vi "Write Data to HW.vi"(11 "CD in":refnum<class "Template.lvclass">) -> (0 "error out":errorcluster, 3 "CD out":refnum<class "Template.lvclass">)   [LabVIEW 2026, in "Template Plugin.lvlib" / "Template.lvclass"]
uses:
  Template.lvclass
  Template.lvclass/Template.ctl
  <userlib>/CustomDeviceInterfaces_v1.lvlibp/custom-device-express-framework/Source/Custom Device Interfaces/CustomDeviceAPI/CustomDeviceAPI.lvclass
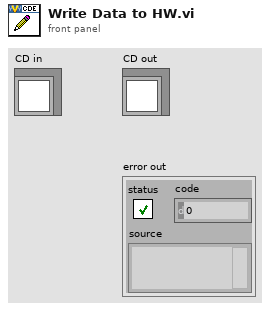
[diagram p1: front panel]
types:
  T1 = cluster{"Data Reference":i32, "Offset":u64, "Length":u64}[]
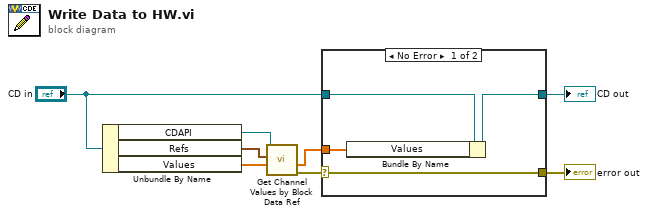
[diagram p0: block diagram]
diagram:
  n1 = Unbundle By Name("CD in") -> ("CDAPI"=w3:refnum<class "CustomDeviceAPI.lvclass">, "Refs"=w2:T1, "Values"=w1:dbl[])
  n2 = call-dynamic "Get Channel Values by Block Data Ref.vi"("Values in"=w1, "Block Data Ref in"=w2, "iCDAPI in"=w3) -> ("error out"=w5:errorcluster, "Values out"=w4:dbl[])  [unwired: 5 in, 2 out]
  n3 = case shown="No Error" w5 {
    selector: w5 -> [w9 w13]
    tunnel: w4 -> [w10 _]
    tunnel: "CD in" -> [w12 w14]
    tunnel: [w11 w14] -> w6
    tunnel: [w9 w13] -> w7
    frame No Error {
      n4 = Bundle By Name(cluster=w12, "Values"=w10) -> (w11:refnum<class "Template.lvclass">)
    }
    frame Error {
    }
  }
  "error out" <- w7
  "CD out" <- w6
